vi "FSIS_MAIN.vi"() -> ()   [LabVIEW 2016]
uses:
  <vilib>/FPGAPlugInAG/cRIO-9067/niLvFpga_Open_cRIO-9067.vi
  <vilib>/rvi/interface/common/dynamic/niFpgaDynamicAddResources.vi
  <vilib>/FPGAPlugInAG/Dynamic/niLvFpga_Run_Dynamic.vi
  <vilib>/Utility/file.llb/Read Delimited Spreadsheet (string).vi
  <vilib>/Utility/error.llb/Error Cluster From Error Code.vi
  <vilib>/rvi/errors/niLvFpgaAdjustHostInterfaceError.vi
  <vilib>/FPGAPlugInAG/Dynamic/niLvFpga_Close_Dynamic.vi
  <vilib>/rvi/interface/nirviOpenFPGA/nirviOpenFPGA.xnode
  FPGA Bitfiles/LabVIEWFPGAtests_FPGATarget_SSFPGADrop1_0hIPb3YkEpA.lvbitx
  SS_FPGA_Drop1.vi
  <vilib>/rvi/interface/nirviMethod/nirviMethod.xnode
  <vilib>/rvi/interface/nirviReadWriteControl/nirviReadWriteControl.xnode
  <vilib>/rvi/interface/nirviCloseFPGA/nirviCloseFPGA.xnode
  <vilib>/rvi/interface/Simulation/niFpgaSimulationCallBeginRW.vi
  NiFpgaLv.dll
panel:
  in  "Tab Control":T1(tab)=enum."OPC UA Server"
  in  "millisecond multiple":u32=1000
  in  "INIT Cluster":T2={"Drop1 Address"="172.22.11.2", "Setup FIle Directory"=path "C:/Users/dhomf/Desktop/Schedules/INI_Files", "System"="SS"}
  out "Flow \nMonitoring\nError":errorcluster
  out "Flow Information":T3(array[cluster])=[{"ID"=193, "Channel Information"="SS_2_6_00__COOL_SBF_01", "Channel Name"="1", "Available Flow"=33.2, "No Operations"=25.0, "Good to Operate"=30.0, "M"=193.0, "c"=-10.0}, {"ID"=195, "Channel Information"="SS_2_6_02__COOL_G1F_01", "Channel Name"="1", "Available Flow"=26.5, "No Operations"=20.0, "Good to Operate"=25.0, "M"=195.0, "c"=-10.0}, {"ID"=197, "Channel Information"="SS_2_6_04__COOL_G2F_01", "Channel Name"="1", "Available Flow"=26.5, "No Operations"=15.0, "Good to Operate"=20.0, "M"=197.0, "c"=-10.0}, {"ID"=199, "Channel Information"="SS_2_6_06__COOL_G3F_01", "Channel Name"="1", "Available Flow"=26.5, "No Operations"=20.0, "Good to Operate"=25.0, "M"=199.0, "c"=-10.0}, {"ID"=201, "Channel Information"="SS_2_6_08__COOL_G4F_01", "Channel Name"="1", "Available Flow"=26.5, "No Operations"=20.0, "Good to Operate"=25.0, "M"=201.0, "c"=-10.0}, {"ID"=203, "Channel Information"="SS_2_6_10__COOL_2NF_01", "Channel Name"="1", "Available Flow"=50.5, "No Operations"=38.0, "Good to Operate"=45.0, "M"=203.0, "c"=-10.0}, {"ID"=205, "Channel Information"="SS_2_6_12__COOL_PBF_01", "Channel Name"="1", "Available Flow"=60.0, "No Operations"=52.0, "Good to Operate"=60.0, "M"=205.0, "c"=-25.0}, {"ID"=207, "Channel Information"="SS_2_6_14__COOL_DSF_01", "Channel Name"="1", "Available Flow"=13.8, "No Operations"=10.0, "Good to Operate"=15.0, "M"=207.0, "c"=-10.0}, {"ID"=209, "Channel Information"="SS_2_7_00__COOL_TRF_01", "Channel Name"="1", "Available Flow"=12.0, "No Operations"=8.0, "Good to Operate"=12.0, "M"=209.0, "c"=-10.0}, {"ID"=211, "Channel Information"="SS_2_7_02__COOL_BCF_01", "Channel Name"="1", "Available Flow"=20.5, "No Operations"=12.0, "Good to Operate"=18.0, "M"=211.0, "c"=-10.0}, {"ID"=213, "Channel Information"="SS_2_7_04__COOL_BPF_01", "Channel Name"="1", "Available Flow"=12.0, "No Operations"=8.0, "Good to Operate"=12.0, "M"=213.0, "c"=-10.0}, {"ID"=215, "Channel Information"="SS_2_7_06__COOL_GBF_01", "Channel Name"="1", "Available Flow"=13.8, "No Operations"=8.0, "Good to Operate"=12.0, "M"=215.0, "c"=-10.0}, {"ID"=217, "Channel Information"="SS_2_7_08__COOL_GCF_01", "Channel Name"="1", "Available Flow"=13.8, "No Operations"=8.0, "Good to Operate"=12.0, "M"=217.0, "c"=-10.0}, {"ID"=219, "Channel Information"="SS_2_7_10__COOL_ISF_01", "Channel Name"="1", "Available Flow"=13.8, "No Operations"=10.0, "Good to Operate"=15.0, "M"=219.0, "c"=-10.0}, {"ID"=221, "Channel Information"="SS_2_7_12__COOL_FRF_01", "Channel Name"="1", "Available Flow"=666.0, "No Operations"=540.0, "Good to Operate"=600.0, "M"=221.0, "c"=-298.80478}, {"ID"=222, "Channel Information"="SS_2_7_13__COOL_FEF_01", "Channel Name"="1", "Available Flow"=1350.0, "No Operations"=1250.0, "Good to Operate"=1350.0, "M"=222.0, "c"=-1363.63636}, {"ID"=223, "Channel Information"="SS_2_7_14__COOL_CAF_01", "Channel Name"="1", "Available Flow"=1500.0, "No Operations"=1380.0, "Good to Operate"=1500.0, "M"=223.0, "c"=-1363.63636}]
  out "FPGA Drop1 Reference Error":errorcluster
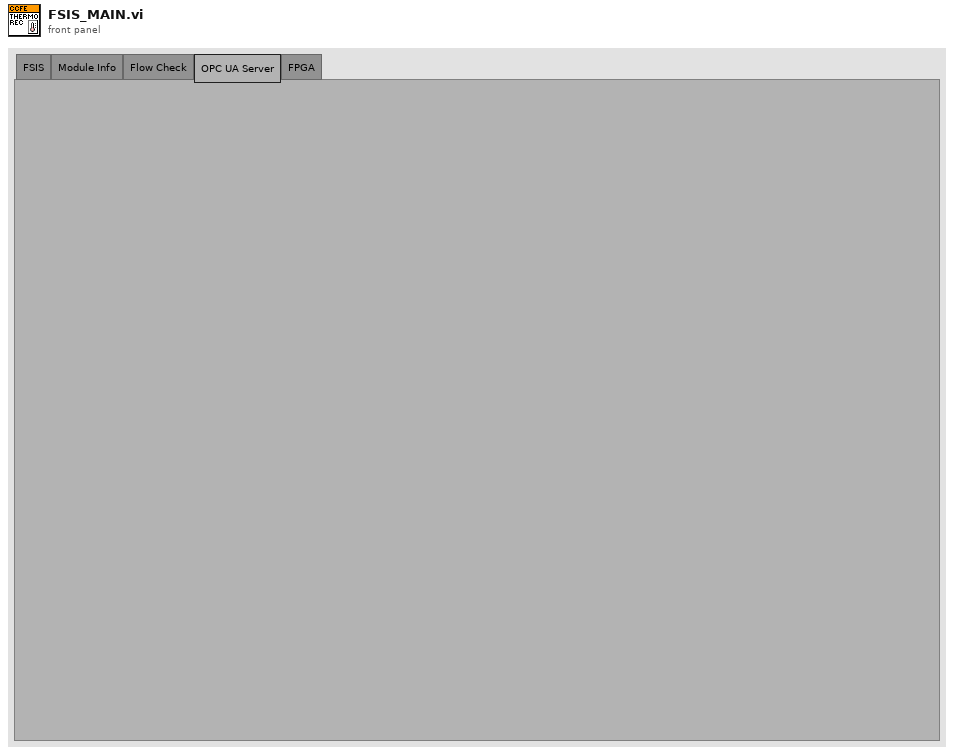
[diagram p1: front panel]
types:
  T1 = enum32{"FSIS", "Module Info", "Flow Check", "OPC UA Server", "FPGA"}
  T2 = cluster{"Drop1 Address":string, "Setup FIle Directory":path, "System":string}
  T3 = cluster{"ID":i32, "Channel Information":string, "Channel Name":string, "Available Flow":dbl, "No Operations":dbl, "Good to Operate":dbl, "M":dbl, "c":dbl}[]
  T4 = cluster{"ID":i32, "Channel Information":string, "Channel Name":string, "Available Flow":dbl, "No Operations":dbl, "Good to Operate":dbl, "M":dbl, "c":dbl}
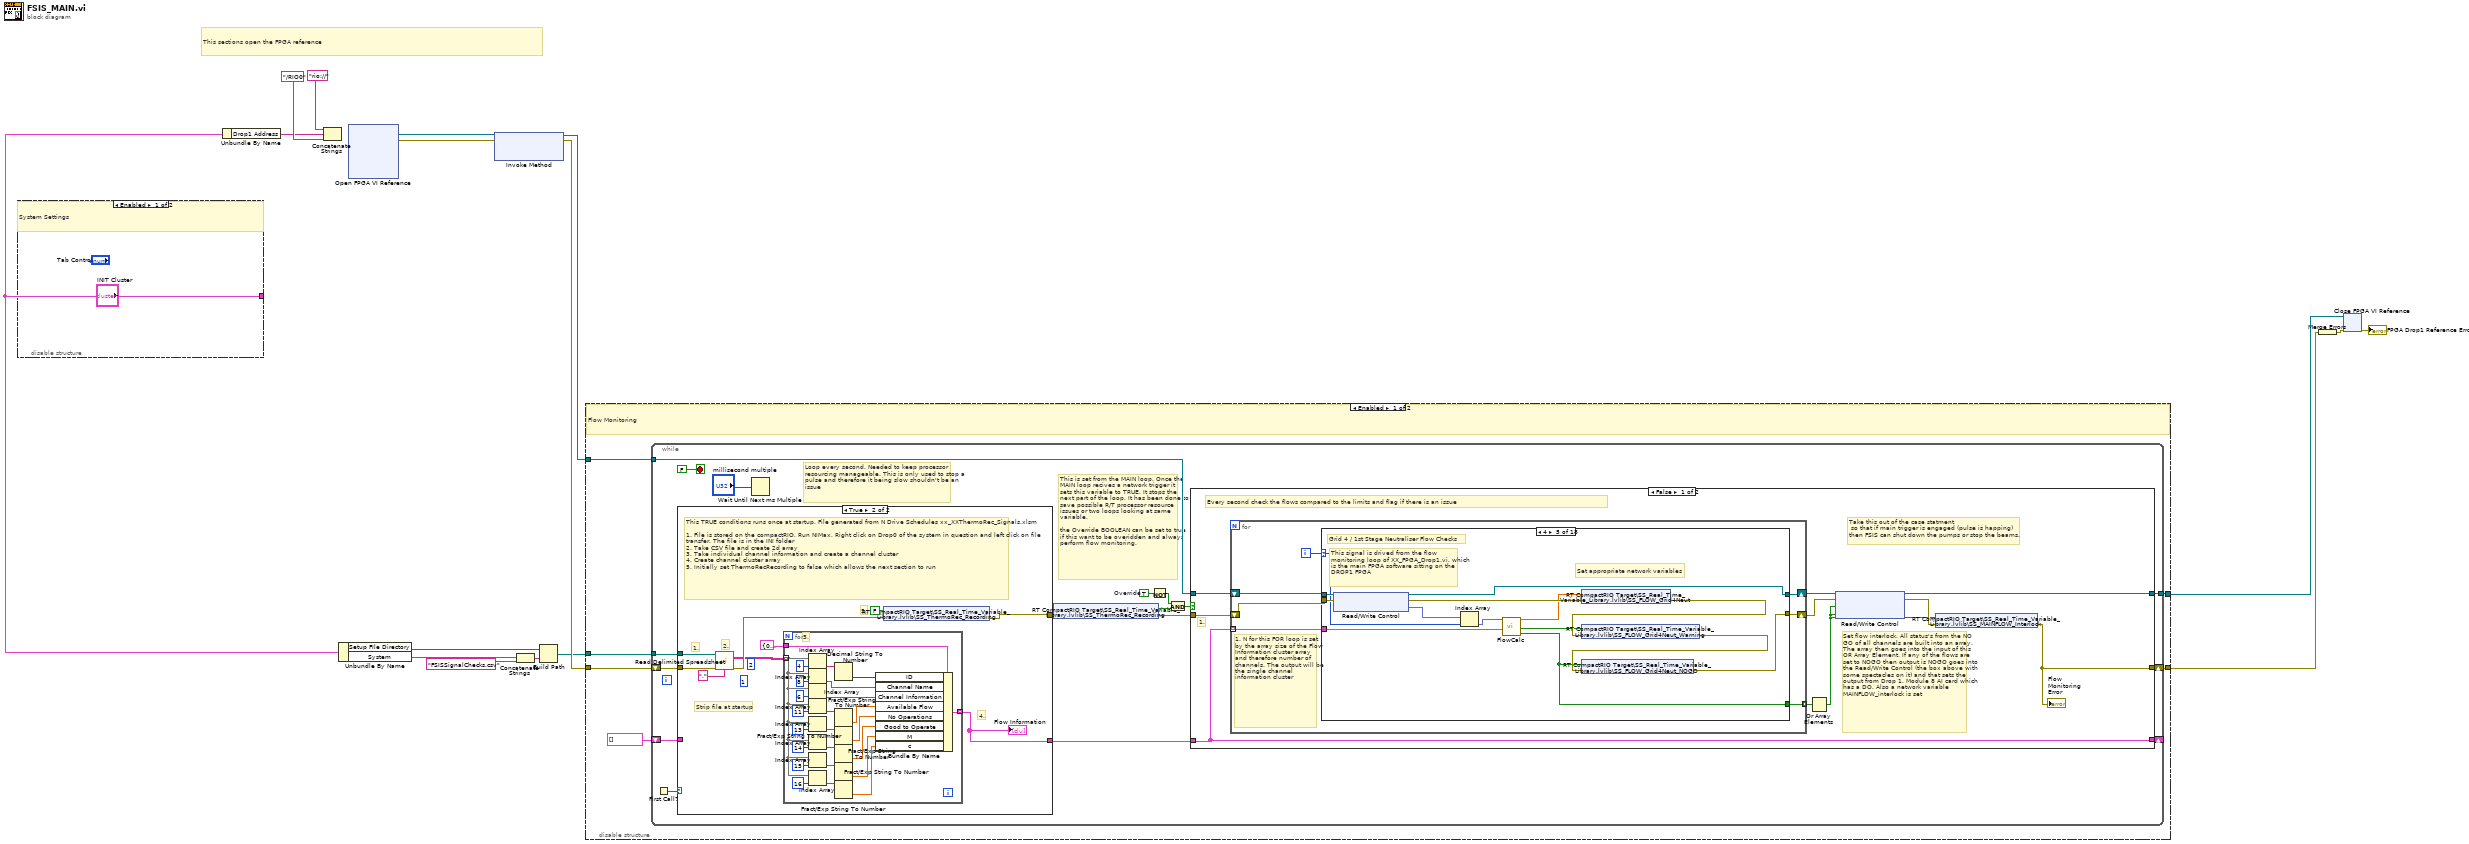
[diagram p0: block diagram]
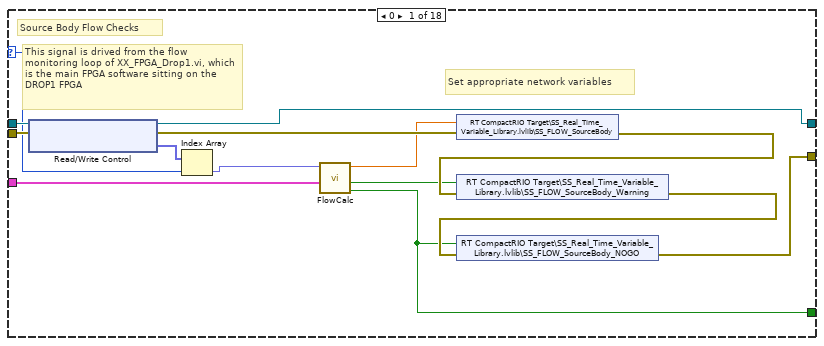
[diagram p3: hidden frame]
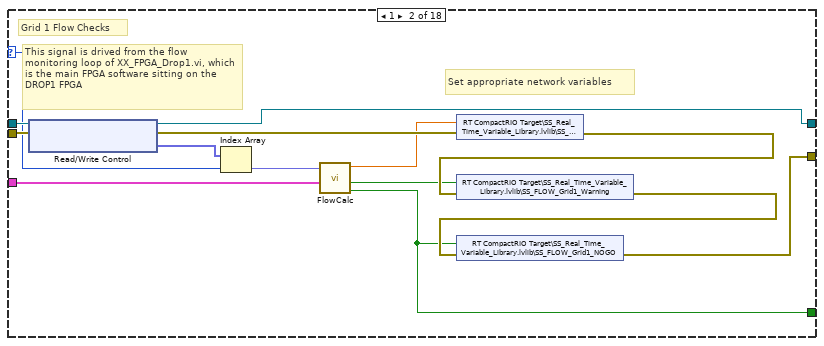
[diagram p4: hidden frame]
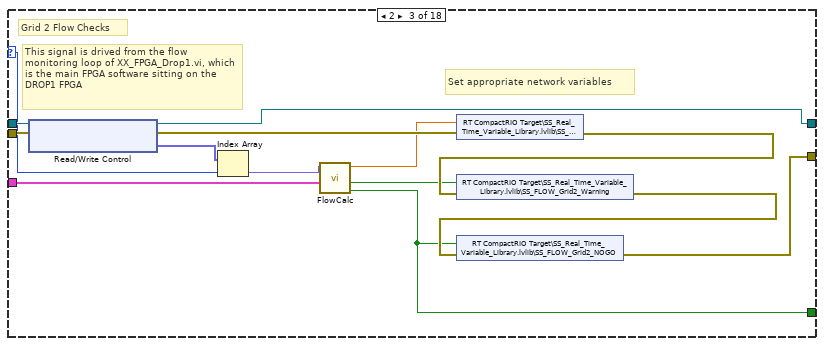
[diagram p5: hidden frame]
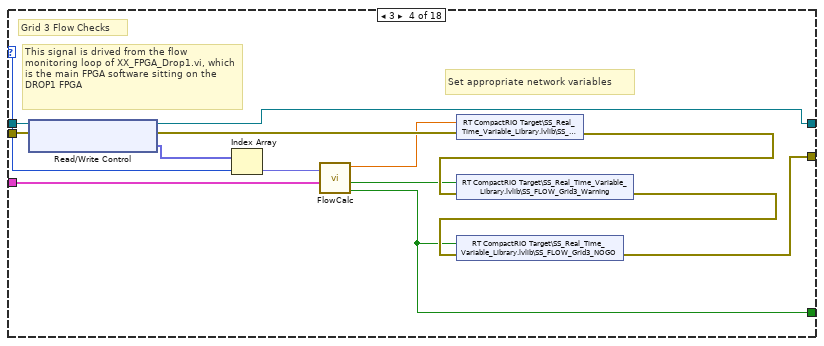
[diagram p6: hidden frame]
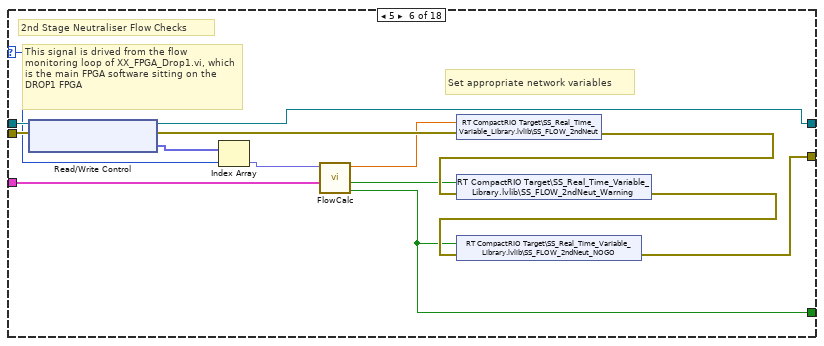
[diagram p7: hidden frame]
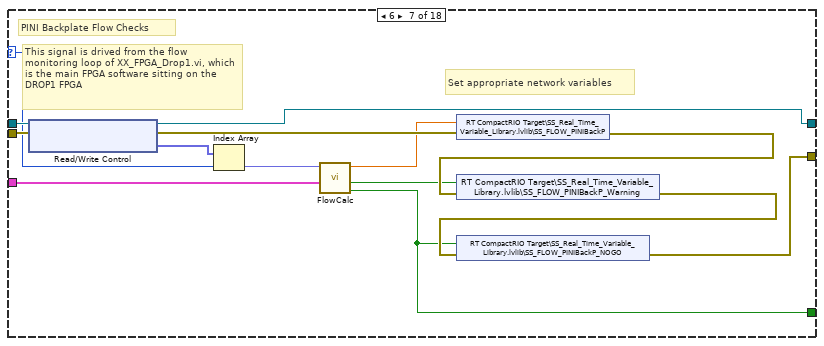
[diagram p8: hidden frame]
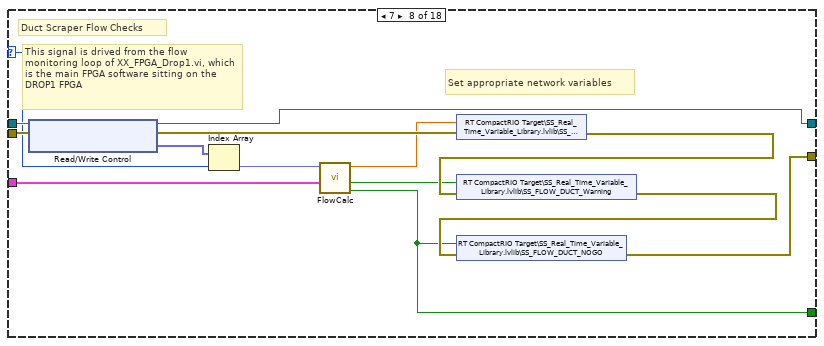
[diagram p9: hidden frame]
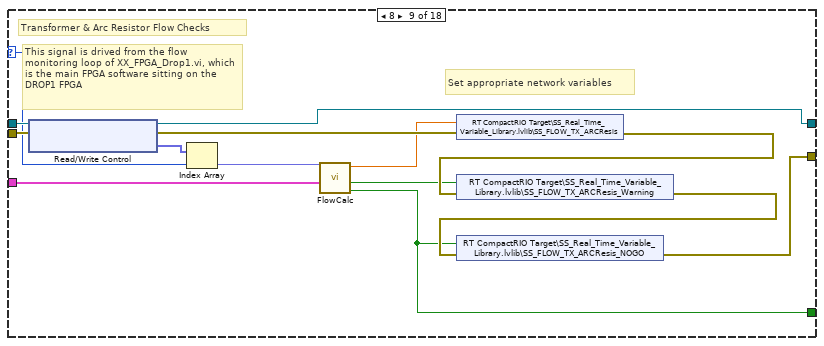
[diagram p10: hidden frame]
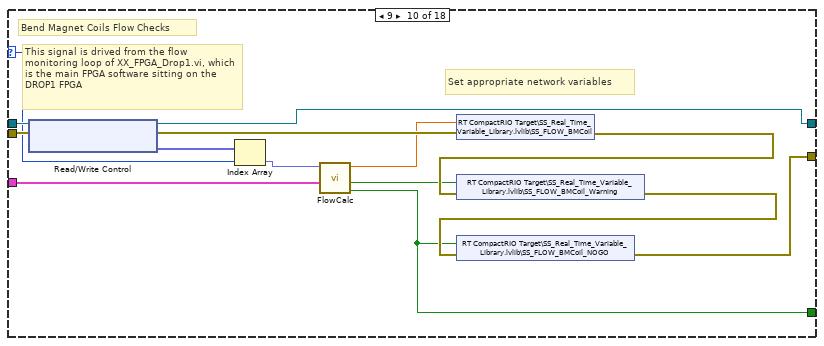
[diagram p11: hidden frame]
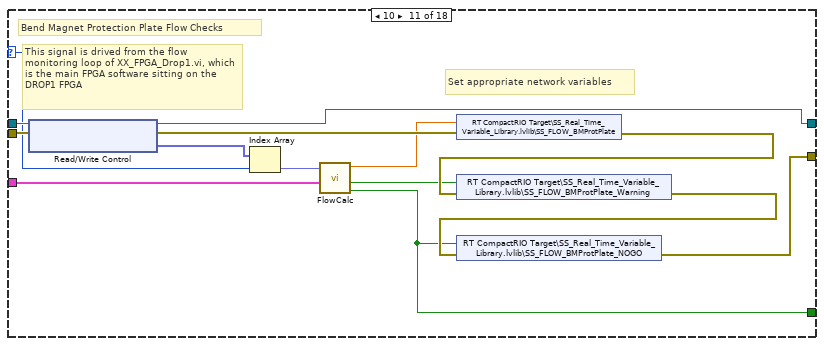
[diagram p12: hidden frame]
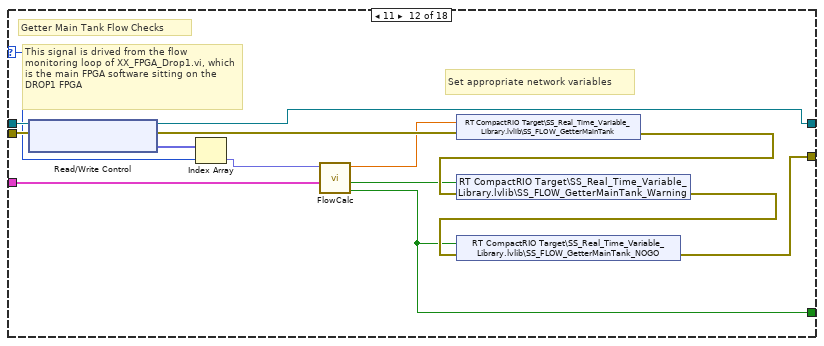
[diagram p13: hidden frame]
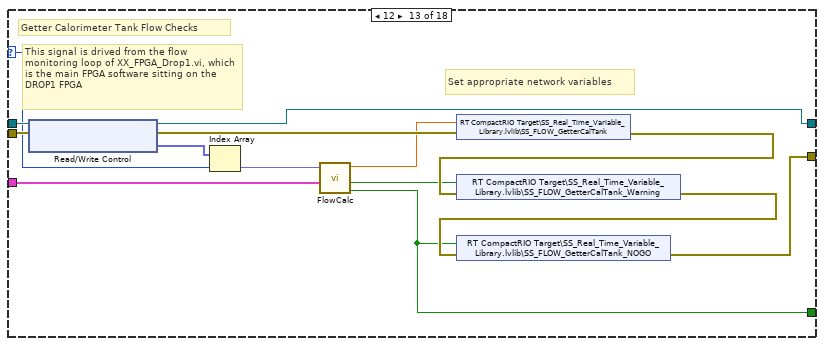
[diagram p14: hidden frame]
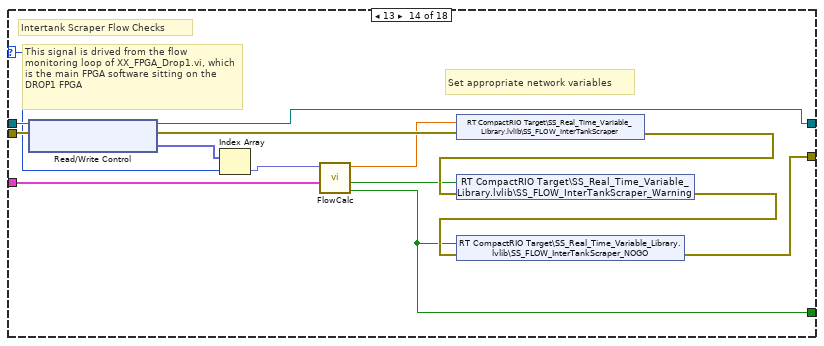
[diagram p15: hidden frame]
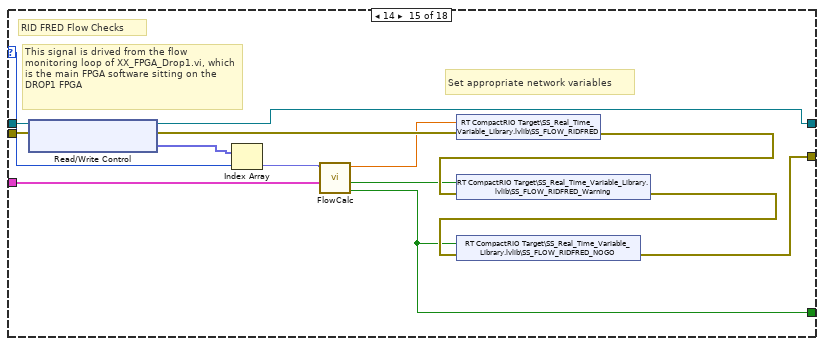
[diagram p16: hidden frame]
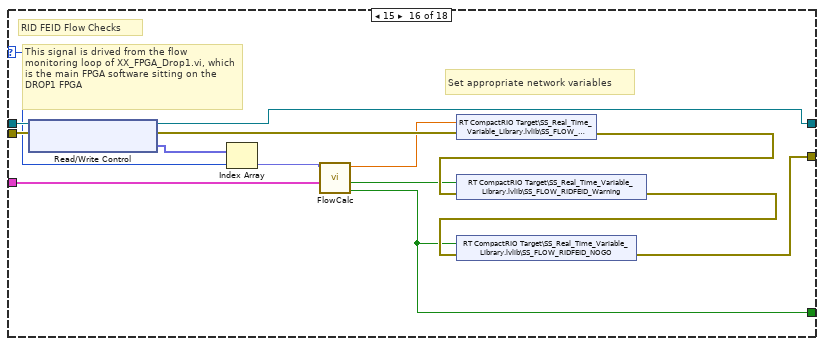
[diagram p17: hidden frame]
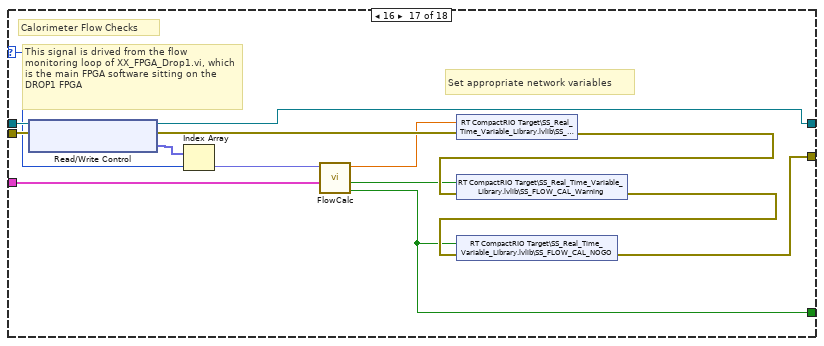
[diagram p18: hidden frame]
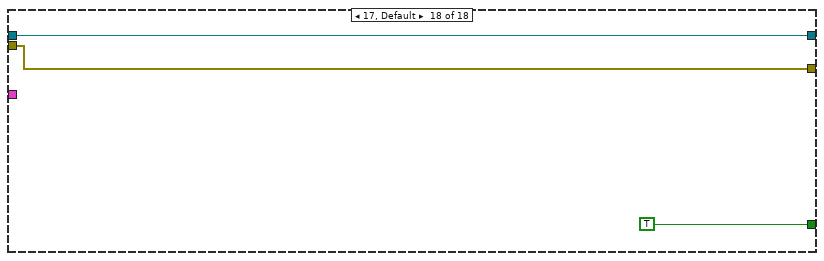
[diagram p19: hidden frame]
diagram:
  # "This sections open the FPGA reference"
  n1 = disable-structure shown="Enabled" {
    disable-tunnel: ["INIT Cluster" _] -> w1
    frame Enabled {
      # "System Settings"
    }
    frame Disabled {
    }
  }
  n2 = Unbundle By Name(w1) -> ("Drop1 Address"=w2:string)
  n3 = Concatenate Strings("rio://", w2, "/RIO0") -> ()  [unwired: 1 out]
  n4 = Unbundle By Name(w1) -> ("Setup FIle Directory"=w4:path, "System"=w3:string)
  n5 = xnode "Open FPGA VI Reference"() -> ("FPGA VI Reference Out"=w14:refnum<k20>, "error out"=w13:errorcluster)  [unwired: 2 in]
  n6 = xnode "Invoke Method"("FPGA VI Reference In"=w14, "error in"=w13) -> ("FPGA VI Reference Out"=w12:refnum<k20>, "error out"=w11:errorcluster)  [unwired: 1 in]
  n7 = Concatenate Strings(w3, "FSISSignalChecks.csv") -> (w7:string)
  n8 = Build Path(base path=w4, name or relative path=w7) -> (appended path=w5:path)
  n9 = disable-structure shown="Enabled" {
    disable-tunnel: [w24 w340] -> w17
    disable-tunnel: w12 -> [w22 w340]
    disable-tunnel: w11 -> [w21 w339]
    disable-tunnel: w5 -> [w20 _]
    disable-tunnel: [w19 w339] -> w8
    frame Enabled {
      # "Flow Monitoring"
      n10 = while {
        shift-right: [w38] -> _
        shift-left: T3 [] ("Flow Information 2") -> [w40]
        tunnel: w22 -> [w36]
        tunnel: [w32] -> w24
        tunnel: w20 -> [w27]
        shift-right: [w26] -> w19
        shift-left: w21 -> [w34]
        stop <- FALSE stop-if-true
        w30 = TRUE  # Override
        # "This is set from the MAIN loop. Once the MAIN loop recives a network trigger it sets this variable to TRUE. It stops the next part of the loop. It has been done to save possible R/T processor resource issues or two loops looking at same variable. \n\nthe Override BOOLEAN can be set to true if this want to be overidden and always perform flow monitoring."
        # "Loop every second. Needed to keep processor resourcing manageable. This is only used to stop a pulse and therefore it being slow shouldn't be an issue"
        # "Flow Monitoring"
        n11 = First Call?() -> (First Call?: T/F=w41:bool)
        n12 = case shown="True" w41 {
          tunnel: w40 -> [w304 _]
          tunnel: [w304 w312] -> w37
          tunnel: w34 -> [w303 w307]
          tunnel: [w303 w308] -> w33
          tunnel: w27 -> [_ w306]
          frame False {
            # "This is the normal situation (after the first loop after startup).  This just passes the information through the FALSE case"
          }
          frame True {
            (unwired) 1 ("index (row)")
            (unwired) 2 ("length")
            # "1."
            # "5."
            # "4."
            # "2."
            # "This TRUE conditions runs once at startup. File generated from N Drive Schedules xx_XXThermoRec_Signals.xlsm\n\n1. File is stored on the compactRIO. Run NIMax, Right click on Drop0 of the system in question and left click on file transfer. The file is in the INI folder\n2. Take CSV file and create 2d array\n3. Take individual channel information and create a channel cluster \n4. Create channel cluster array\n5. Initially set ThermoRecRecording to false which allows the next section to run"
            # "Strip file at startup"
            n13 = call-poly <vilib>:"Read Delimited Spreadsheet.vi"("file path (dialog if empty)"=w306, "error in (no error)"=w307, "delimiter (\\t)"="," ("delimiter (\\t)")) -> ("all rows"=w305:string[][], "error out"=w309:errorcluster)  [unwired: 7 in, 4 out]
            n14 = for {
              tunnel: w305 -> [w317] mode=indexing
              tunnel: T4 {"ID"=0, "Channel Information"="", "Channel Name"="", "Available Flow"=0.0, "No Operations"=0.0, "Good to Operate"=0.0, "M"=0.0, "c"=0.0} ("Flow Information 2") -> [w338]
              tunnel: [w321] -> w312 mode=indexing
              # "3."
              n15 = Index Array(array=w317, index=4) -> (element=w336:string)
              n16 = Index Array(array=w317, index=8) -> (element=w329:string)
              n17 = Index Array(array=w317, index=6) -> (element=w328:string)
              n18 = Index Array(array=w317, index=11) -> (element=w327:string)
              n19 = Index Array(array=w317, index=13) -> (element=w323:string)
              n20 = Index Array(array=w317, index=14) -> (element=w322:string)
              n21 = Index Array(array=w317, index=15) -> (element=w319:string)
              n22 = Index Array(array=w317, index=16) -> (element=w320:string)
              n23 = Fract/Exp String To Number(string=w327) -> (number=w326:dbl)  [unwired: 3 in, 1 out]
              n24 = Fract/Exp String To Number(string=w323) -> (number=w325:dbl)  [unwired: 3 in, 1 out]
              n25 = Fract/Exp String To Number(string=w322) -> (number=w324:dbl)  [unwired: 3 in, 1 out]
              n26 = Fract/Exp String To Number(string=w319) -> (number=w316:dbl)  [unwired: 3 in, 1 out]
              n27 = Fract/Exp String To Number(string=w320) -> (number=w315:dbl)  [unwired: 3 in, 1 out]
              n28 = Decimal String To Number(string=w336) -> (number=w335:i32)  [unwired: 2 in, 1 out]
              n29 = Bundle By Name(cluster=w338, "ID"=w335, "Channel Name"=w329, "Channel Information"=w328, "Available Flow"=w326, "No Operations"=w325, "Good to Operate"=w324, "M"=w316, "c"=w315) -> (w321:T4)
            }
            "Flow Information" <- w312
            n30 = shared-variable "RT CompactRIO Target\\SS_Real_Time_Variable_Library.lvlib\\SS_ThermoRec_Recording"(FALSE ("SS_ThermoRec_Recording"), error in=w309) -> (error out=w308:errorcluster)
          }
        }
        n31 = Wait Until Next ms Multiple(millisecond multiple="millisecond multiple") -> ()  [unwired: 1 out]
        n32 = shared-variable "RT CompactRIO Target\\SS_Real_Time_Variable_Library.lvlib\\SS_ThermoRec_Recording"(error in=w33) -> (w28:bool, error out=w35:errorcluster)
        n33 = Not(x=w30) -> (.not. x?=w31:bool)
        n34 = And(x=w31, y=w28) -> (x .and. y?=w29:bool)
        n35 = case shown="False" w29 {
          tunnel: w37 -> [w45 w302]
          tunnel: [w45 w302] -> w38
          tunnel: w36 -> [w51 w301]
          tunnel: w35 -> [w50 w300]
          tunnel: [w46 w301] -> w32
          tunnel: [w43 w300] -> w26
          frame False {
            # "Take this out of the case statment\n so that if main trigger is engaged (pulse is happing) \nthen FSIS can shut down the pumps or stop the beams."
            # "Set flow interlock. All status's from the NO GO of all channels are built into an array. The array then goes into the input of this OR Array Element. If any of the flows are set to NOGO then output is NOGO goes into the Read/Write Control (the box above with some spectacles on it) and that sets the output from Drop 1, Module 8 AI card which has a DO. Also a network variable MAINFLOW_interlock is set"
            # "1."
            # "Every second check the flows compared to the limits and flag if there is an issue"
            n36 = for {
              tunnel: w45 -> [w52] mode=indexing
              shift-right: [w54] -> w47
              shift-left: w50 -> [w56]
              shift-right: [w55] -> w48
              shift-left: w51 -> [w57]
              tunnel: [w53] -> w49 mode=indexing
              i -> [w58]
              # "1. N for this FOR loop is set by the array size of the Flow Information cluster array and therefore number of channels. The output will be the single channel information cluster"
              n37 = case shown="4" w58 {
                selector: w58 -> [w60 w74 w88 w102 w116 w130 w144 w158 w171 w185 w199 w213 w227 w241 w256 w270 w284 _]
                tunnel: w57 -> [w72 w86 w100 w114 w128 w142 w156 w170 w184 w198 w212 w226 w240 w254 w268 w282 w296 w298]
                tunnel: w56 -> [w71 w85 w99 w113 w127 w141 w155 w169 w183 w197 w211 w225 w239 w253 w267 w281 w295 w299]
                tunnel: [w66 w80 w94 w108 w122 w136 w150 w164 w178 w192 w206 w220 w234 w248 w262 w276 w290 w298] -> w55
                tunnel: [w69 w83 w97 w111 w125 w139 w153 w167 w181 w195 w209 w223 w237 w251 w265 w279 w293 w299] -> w54
                tunnel: [w63 w77 w91 w105 w119 w133 w147 w161 w175 w189 w203 w217 w231 w245 w259 w273 w287 TRUE] -> w53
                tunnel: w52 -> [w65 w79 w93 w107 w121 w135 w149 w163 w177 w191 w205 w219 w233 w247 w261 w275 w289 _]
                frame 0 {
                  # "Set appropriate network variables"
                  # "This signal is drived from the flow monitoring loop of XX_FPGA_Drop1.vi, which is the main FPGA software sitting on the DROP1 FPGA"
                  # "Source Body Flow Checks"
                  n38 = xnode "Read/Write Control"("FPGA VI Reference In"=w72, "error in"=w71) -> ("FPGA VI Reference Out"=w66:refnum<k20>, "error out"=w70:errorcluster, "Raw Data out Mod 1"=w61:fxp<+/-,24,-4>[])
                  n39 = Index Array(array=w61, index=w60) -> (element=w59:fxp<+/-,24,-4>)
                  n40 = call "FlowCalc.vi"("Individual Channel Cluster"=w65, "Flow"=w59) -> ("Flow - No Operations"=w63:bool, "Flow - Warning"=w62:bool, "Flow Rate"=w64:dbl)  [unwired: 7 in]
                  n41 = shared-variable "RT CompactRIO Target\\SS_Real_Time_Variable_Library.lvlib\\SS_FLOW_SourceBody"(w64, error in=w70) -> (error out=w67:errorcluster)
                  n42 = shared-variable "RT CompactRIO Target\\SS_Real_Time_Variable_Library.lvlib\\SS_FLOW_SourceBody_Warning"(w62, error in=w67) -> (error out=w68:errorcluster)
                  n43 = shared-variable "RT CompactRIO Target\\SS_Real_Time_Variable_Library.lvlib\\SS_FLOW_SourceBody_NOGO"(w63, error in=w68) -> (error out=w69:errorcluster)
                }
                frame 1 {
                  # "Grid 1 Flow Checks"
                  # "Set appropriate network variables"
                  # "This signal is drived from the flow monitoring loop of XX_FPGA_Drop1.vi, which is the main FPGA software sitting on the DROP1 FPGA"
                  n44 = xnode "Read/Write Control"("FPGA VI Reference In"=w86, "error in"=w85) -> ("FPGA VI Reference Out"=w80:refnum<k20>, "error out"=w84:errorcluster, "Raw Data out Mod 1"=w75:fxp<+/-,24,-4>[])
                  n45 = Index Array(array=w75, index=w74) -> (element=w73:fxp<+/-,24,-4>)
                  n46 = call "FlowCalc.vi"("Individual Channel Cluster"=w79, "Flow"=w73) -> ("Flow - No Operations"=w77:bool, "Flow - Warning"=w76:bool, "Flow Rate"=w78:dbl)  [unwired: 7 in]
                  n47 = shared-variable "RT CompactRIO Target\\SS_Real_Time_Variable_Library.lvlib\\SS_FLOW_Grid1"(w78, error in=w84) -> (error out=w81:errorcluster)
                  n48 = shared-variable "RT CompactRIO Target\\SS_Real_Time_Variable_Library.lvlib\\SS_FLOW_Grid1_Warning"(w76, error in=w81) -> (error out=w82:errorcluster)
                  n49 = shared-variable "RT CompactRIO Target\\SS_Real_Time_Variable_Library.lvlib\\SS_FLOW_Grid1_NOGO"(w77, error in=w82) -> (error out=w83:errorcluster)
                }
                frame 2 {
                  # "Grid 2 Flow Checks"
                  # "Set appropriate network variables"
                  # "This signal is drived from the flow monitoring loop of XX_FPGA_Drop1.vi, which is the main FPGA software sitting on the DROP1 FPGA"
                  n50 = xnode "Read/Write Control"("FPGA VI Reference In"=w100, "error in"=w99) -> ("FPGA VI Reference Out"=w94:refnum<k20>, "error out"=w98:errorcluster, "Raw Data out Mod 1"=w89:fxp<+/-,24,-4>[])
                  n51 = Index Array(array=w89, index=w88) -> (element=w87:fxp<+/-,24,-4>)
                  n52 = call "FlowCalc.vi"("Individual Channel Cluster"=w93, "Flow"=w87) -> ("Flow - No Operations"=w91:bool, "Flow - Warning"=w90:bool, "Flow Rate"=w92:dbl)  [unwired: 7 in]
                  n53 = shared-variable "RT CompactRIO Target\\SS_Real_Time_Variable_Library.lvlib\\SS_FLOW_Grid2"(w92, error in=w98) -> (error out=w95:errorcluster)
                  n54 = shared-variable "RT CompactRIO Target\\SS_Real_Time_Variable_Library.lvlib\\SS_FLOW_Grid2_Warning"(w90, error in=w95) -> (error out=w96:errorcluster)
                  n55 = shared-variable "RT CompactRIO Target\\SS_Real_Time_Variable_Library.lvlib\\SS_FLOW_Grid2_NOGO"(w91, error in=w96) -> (error out=w97:errorcluster)
                }
                frame 3 {
                  # "Grid 3 Flow Checks"
                  # "Set appropriate network variables"
                  # "This signal is drived from the flow monitoring loop of XX_FPGA_Drop1.vi, which is the main FPGA software sitting on the DROP1 FPGA"
                  n56 = xnode "Read/Write Control"("FPGA VI Reference In"=w114, "error in"=w113) -> ("FPGA VI Reference Out"=w108:refnum<k20>, "error out"=w112:errorcluster, "Raw Data out Mod 1"=w103:fxp<+/-,24,-4>[])
                  n57 = Index Array(array=w103, index=w102) -> (element=w101:fxp<+/-,24,-4>)
                  n58 = call "FlowCalc.vi"("Individual Channel Cluster"=w107, "Flow"=w101) -> ("Flow - No Operations"=w105:bool, "Flow - Warning"=w104:bool, "Flow Rate"=w106:dbl)  [unwired: 7 in]
                  n59 = shared-variable "RT CompactRIO Target\\SS_Real_Time_Variable_Library.lvlib\\SS_FLOW_Grid3"(w106, error in=w112) -> (error out=w109:errorcluster)
                  n60 = shared-variable "RT CompactRIO Target\\SS_Real_Time_Variable_Library.lvlib\\SS_FLOW_Grid3_Warning"(w104, error in=w109) -> (error out=w110:errorcluster)
                  n61 = shared-variable "RT CompactRIO Target\\SS_Real_Time_Variable_Library.lvlib\\SS_FLOW_Grid3_NOGO"(w105, error in=w110) -> (error out=w111:errorcluster)
                }
                frame 4 {
                  # "Grid 4 / 1st Stage Neutraliser Flow Checks"
                  # "Set appropriate network variables"
                  # "This signal is drived from the flow monitoring loop of XX_FPGA_Drop1.vi, which is the main FPGA software sitting on the DROP1 FPGA"
                  n62 = xnode "Read/Write Control"("FPGA VI Reference In"=w128, "error in"=w127) -> ("FPGA VI Reference Out"=w122:refnum<k20>, "error out"=w126:errorcluster, "Raw Data out Mod 1"=w117:fxp<+/-,24,-4>[])
                  n63 = Index Array(array=w117, index=w116) -> (element=w115:fxp<+/-,24,-4>)
                  n64 = call "FlowCalc.vi"("Individual Channel Cluster"=w121, "Flow"=w115) -> ("Flow - No Operations"=w119:bool, "Flow - Warning"=w118:bool, "Flow Rate"=w120:dbl)  [unwired: 7 in]
                  n65 = shared-variable "RT CompactRIO Target\\SS_Real_Time_Variable_Library.lvlib\\SS_FLOW_Grid4Neut"(w120, error in=w126) -> (error out=w123:errorcluster)
                  n66 = shared-variable "RT CompactRIO Target\\SS_Real_Time_Variable_Library.lvlib\\SS_FLOW_Grid4Neut_Warning"(w118, error in=w123) -> (error out=w124:errorcluster)
                  n67 = shared-variable "RT CompactRIO Target\\SS_Real_Time_Variable_Library.lvlib\\SS_FLOW_Grid4Neut_NOGO"(w119, error in=w124) -> (error out=w125:errorcluster)
                }
                frame 5 {
                  # "2nd Stage Neutraliser Flow Checks"
                  # "Set appropriate network variables"
                  # "This signal is drived from the flow monitoring loop of XX_FPGA_Drop1.vi, which is the main FPGA software sitting on the DROP1 FPGA"
                  n68 = xnode "Read/Write Control"("FPGA VI Reference In"=w142, "error in"=w141) -> ("FPGA VI Reference Out"=w136:refnum<k20>, "error out"=w140:errorcluster, "Raw Data out Mod 1"=w131:fxp<+/-,24,-4>[])
                  n69 = Index Array(array=w131, index=w130) -> (element=w129:fxp<+/-,24,-4>)
                  n70 = call "FlowCalc.vi"("Individual Channel Cluster"=w135, "Flow"=w129) -> ("Flow - No Operations"=w133:bool, "Flow - Warning"=w132:bool, "Flow Rate"=w134:dbl)  [unwired: 7 in]
                  n71 = shared-variable "RT CompactRIO Target\\SS_Real_Time_Variable_Library.lvlib\\SS_FLOW_2ndNeut"(w134, error in=w140) -> (error out=w137:errorcluster)
                  n72 = shared-variable "RT CompactRIO Target\\SS_Real_Time_Variable_Library.lvlib\\SS_FLOW_2ndNeut_Warning"(w132, error in=w137) -> (error out=w138:errorcluster)
                  n73 = shared-variable "RT CompactRIO Target\\SS_Real_Time_Variable_Library.lvlib\\SS_FLOW_2ndNeut_NOGO"(w133, error in=w138) -> (error out=w139:errorcluster)
                }
                frame 6 {
                  # "PINI Backplate Flow Checks"
                  # "Set appropriate network variables"
                  # "This signal is drived from the flow monitoring loop of XX_FPGA_Drop1.vi, which is the main FPGA software sitting on the DROP1 FPGA"
                  n74 = xnode "Read/Write Control"("FPGA VI Reference In"=w156, "error in"=w155) -> ("FPGA VI Reference Out"=w150:refnum<k20>, "error out"=w154:errorcluster, "Raw Data out Mod 1"=w145:fxp<+/-,24,-4>[])
                  n75 = Index Array(array=w145, index=w144) -> (element=w143:fxp<+/-,24,-4>)
                  n76 = call "FlowCalc.vi"("Individual Channel Cluster"=w149, "Flow"=w143) -> ("Flow - No Operations"=w147:bool, "Flow - Warning"=w146:bool, "Flow Rate"=w148:dbl)  [unwired: 7 in]
                  n77 = shared-variable "RT CompactRIO Target\\SS_Real_Time_Variable_Library.lvlib\\SS_FLOW_PINIBackP"(w148, error in=w154) -> (error out=w151:errorcluster)
                  n78 = shared-variable "RT CompactRIO Target\\SS_Real_Time_Variable_Library.lvlib\\SS_FLOW_PINIBackP_Warning"(w146, error in=w151) -> (error out=w152:errorcluster)
                  n79 = shared-variable "RT CompactRIO Target\\SS_Real_Time_Variable_Library.lvlib\\SS_FLOW_PINIBackP_NOGO"(w147, error in=w152) -> (error out=w153:errorcluster)
                }
                frame 7 {
                  # "Duct Scraper Flow Checks"
                  # "Set appropriate network variables"
                  # "This signal is drived from the flow monitoring loop of XX_FPGA_Drop1.vi, which is the main FPGA software sitting on the DROP1 FPGA"
                  n80 = xnode "Read/Write Control"("FPGA VI Reference In"=w170, "error in"=w169) -> ("FPGA VI Reference Out"=w164:refnum<k20>, "error out"=w168:errorcluster, "Raw Data out Mod 1"=w159:fxp<+/-,24,-4>[])
                  n81 = Index Array(array=w159, index=w158) -> (element=w157:fxp<+/-,24,-4>)
                  n82 = call "FlowCalc.vi"("Individual Channel Cluster"=w163, "Flow"=w157) -> ("Flow - No Operations"=w161:bool, "Flow - Warning"=w160:bool, "Flow Rate"=w162:dbl)  [unwired: 7 in]
                  n83 = shared-variable "RT CompactRIO Target\\SS_Real_Time_Variable_Library.lvlib\\SS_FLOW_DUCT"(w162, error in=w168) -> (error out=w165:errorcluster)
                  n84 = shared-variable "RT CompactRIO Target\\SS_Real_Time_Variable_Library.lvlib\\SS_FLOW_DUCT_Warning"(w160, error in=w165) -> (error out=w166:errorcluster)
                  n85 = shared-variable "RT CompactRIO Target\\SS_Real_Time_Variable_Library.lvlib\\SS_FLOW_DUCT_NOGO"(w161, error in=w166) -> (error out=w167:errorcluster)
                }
                frame 8 {
                  # "Transformer & Arc Resistor Flow Checks"
                  # "Set appropriate network variables"
                  # "This signal is drived from the flow monitoring loop of XX_FPGA_Drop1.vi, which is the main FPGA software sitting on the DROP1 FPGA"
                  n86 = xnode "Read/Write Control"("FPGA VI Reference In"=w184, "error in"=w183) -> ("FPGA VI Reference Out"=w178:refnum<k20>, "error out"=w182:errorcluster, "Raw Data out Mod 1"=w172:fxp<+/-,24,-4>[])
                  n87 = Index Array(array=w172, index=w171) -> (element=w173:fxp<+/-,24,-4>)
                  n88 = call "FlowCalc.vi"("Individual Channel Cluster"=w177, "Flow"=w173) -> ("Flow - No Operations"=w175:bool, "Flow - Warning"=w174:bool, "Flow Rate"=w176:dbl)  [unwired: 7 in]
                  n89 = shared-variable "RT CompactRIO Target\\SS_Real_Time_Variable_Library.lvlib\\SS_FLOW_TX_ARCResis"(w176, error in=w182) -> (error out=w179:errorcluster)
                  n90 = shared-variable "RT CompactRIO Target\\SS_Real_Time_Variable_Library.lvlib\\SS_FLOW_TX_ARCResis_Warning"(w174, error in=w179) -> (error out=w180:errorcluster)
                  n91 = shared-variable "RT CompactRIO Target\\SS_Real_Time_Variable_Library.lvlib\\SS_FLOW_TX_ARCResis_NOGO"(w175, error in=w180) -> (error out=w181:errorcluster)
                }
                frame 9 {
                  # "Bend Magnet Coils Flow Checks"
                  # "Set appropriate network variables"
                  # "This signal is drived from the flow monitoring loop of XX_FPGA_Drop1.vi, which is the main FPGA software sitting on the DROP1 FPGA"
                  n92 = xnode "Read/Write Control"("FPGA VI Reference In"=w198, "error in"=w197) -> ("FPGA VI Reference Out"=w192:refnum<k20>, "error out"=w196:errorcluster, "Raw Data out Mod 1"=w186:fxp<+/-,24,-4>[])
                  n93 = Index Array(array=w186, index=w185) -> (element=w187:fxp<+/-,24,-4>)
                  n94 = call "FlowCalc.vi"("Individual Channel Cluster"=w191, "Flow"=w187) -> ("Flow - No Operations"=w189:bool, "Flow - Warning"=w188:bool, "Flow Rate"=w190:dbl)  [unwired: 7 in]
                  n95 = shared-variable "RT CompactRIO Target\\SS_Real_Time_Variable_Library.lvlib\\SS_FLOW_BMCoil"(w190, error in=w196) -> (error out=w193:errorcluster)
                  n96 = shared-variable "RT CompactRIO Target\\SS_Real_Time_Variable_Library.lvlib\\SS_FLOW_BMCoil_Warning"(w188, error in=w193) -> (error out=w194:errorcluster)
                  n97 = shared-variable "RT CompactRIO Target\\SS_Real_Time_Variable_Library.lvlib\\SS_FLOW_BMCoil_NOGO"(w189, error in=w194) -> (error out=w195:errorcluster)
                }
                frame 10 {
                  # "Bend Magnet Protection Plate Flow Checks"
                  # "Set appropriate network variables"
                  # "This signal is drived from the flow monitoring loop of XX_FPGA_Drop1.vi, which is the main FPGA software sitting on the DROP1 FPGA"
                  n98 = xnode "Read/Write Control"("FPGA VI Reference In"=w212, "error in"=w211) -> ("FPGA VI Reference Out"=w206:refnum<k20>, "error out"=w210:errorcluster, "Raw Data out Mod 1"=w200:fxp<+/-,24,-4>[])
                  n99 = Index Array(array=w200, index=w199) -> (element=w201:fxp<+/-,24,-4>)
                  n100 = call "FlowCalc.vi"("Individual Channel Cluster"=w205, "Flow"=w201) -> ("Flow - No Operations"=w203:bool, "Flow - Warning"=w202:bool, "Flow Rate"=w204:dbl)  [unwired: 7 in]
                  n101 = shared-variable "RT CompactRIO Target\\SS_Real_Time_Variable_Library.lvlib\\SS_FLOW_BMProtPlate"(w204, error in=w210) -> (error out=w207:errorcluster)
                  n102 = shared-variable "RT CompactRIO Target\\SS_Real_Time_Variable_Library.lvlib\\SS_FLOW_BMProtPlate_Warning"(w202, error in=w207) -> (error out=w208:errorcluster)
                  n103 = shared-variable "RT CompactRIO Target\\SS_Real_Time_Variable_Library.lvlib\\SS_FLOW_BMProtPlate_NOGO"(w203, error in=w208) -> (error out=w209:errorcluster)
                }
                frame 11 {
                  # "Getter Main Tank Flow Checks"
                  # "Set appropriate network variables"
                  # "This signal is drived from the flow monitoring loop of XX_FPGA_Drop1.vi, which is the main FPGA software sitting on the DROP1 FPGA"
                  n104 = xnode "Read/Write Control"("FPGA VI Reference In"=w226, "error in"=w225) -> ("FPGA VI Reference Out"=w220:refnum<k20>, "error out"=w224:errorcluster, "Raw Data out Mod 1"=w214:fxp<+/-,24,-4>[])
                  n105 = Index Array(array=w214, index=w213) -> (element=w215:fxp<+/-,24,-4>)
                  n106 = call "FlowCalc.vi"("Individual Channel Cluster"=w219, "Flow"=w215) -> ("Flow - No Operations"=w217:bool, "Flow - Warning"=w216:bool, "Flow Rate"=w218:dbl)  [unwired: 7 in]
                  n107 = shared-variable "RT CompactRIO Target\\SS_Real_Time_Variable_Library.lvlib\\SS_FLOW_GetterMainTank"(w218, error in=w224) -> (error out=w221:errorcluster)
                  n108 = shared-variable "RT CompactRIO Target\\SS_Real_Time_Variable_Library.lvlib\\SS_FLOW_GetterMainTank_Warning"(w216, error in=w221) -> (error out=w222:errorcluster)
                  n109 = shared-variable "RT CompactRIO Target\\SS_Real_Time_Variable_Library.lvlib\\SS_FLOW_GetterMainTank_NOGO"(w217, error in=w222) -> (error out=w223:errorcluster)
                }
                frame 12 {
                  # "Getter Calorimeter Tank Flow Checks"
                  # "Set appropriate network variables"
                  # "This signal is drived from the flow monitoring loop of XX_FPGA_Drop1.vi, which is the main FPGA software sitting on the DROP1 FPGA"
                  n110 = xnode "Read/Write Control"("FPGA VI Reference In"=w240, "error in"=w239) -> ("FPGA VI Reference Out"=w234:refnum<k20>, "error out"=w238:errorcluster, "Raw Data out Mod 1"=w228:fxp<+/-,24,-4>[])
                  n111 = Index Array(array=w228, index=w227) -> (element=w229:fxp<+/-,24,-4>)
                  n112 = call "FlowCalc.vi"("Individual Channel Cluster"=w233, "Flow"=w229) -> ("Flow - No Operations"=w231:bool, "Flow - Warning"=w230:bool, "Flow Rate"=w232:dbl)  [unwired: 7 in]
                  n113 = shared-variable "RT CompactRIO Target\\SS_Real_Time_Variable_Library.lvlib\\SS_FLOW_GetterCalTank"(w232, error in=w238) -> (error out=w235:errorcluster)
                  n114 = shared-variable "RT CompactRIO Target\\SS_Real_Time_Variable_Library.lvlib\\SS_FLOW_GetterCalTank_Warning"(w230, error in=w235) -> (error out=w236:errorcluster)
                  n115 = shared-variable "RT CompactRIO Target\\SS_Real_Time_Variable_Library.lvlib\\SS_FLOW_GetterCalTank_NOGO"(w231, error in=w236) -> (error out=w237:errorcluster)
                }
                frame 13 {
                  # "Intertank Scraper Flow Checks"
                  # "Set appropriate network variables"
                  # "This signal is drived from the flow monitoring loop of XX_FPGA_Drop1.vi, which is the main FPGA software sitting on the DROP1 FPGA"
                  n116 = xnode "Read/Write Control"("FPGA VI Reference In"=w254, "error in"=w253) -> ("FPGA VI Reference Out"=w248:refnum<k20>, "error out"=w252:errorcluster, "Raw Data out Mod 1"=w242:fxp<+/-,24,-4>[])
                  n117 = Index Array(array=w242, index=w241) -> (element=w243:fxp<+/-,24,-4>)
                  n118 = call "FlowCalc.vi"("Individual Channel Cluster"=w247, "Flow"=w243) -> ("Flow - No Operations"=w245:bool, "Flow - Warning"=w244:bool, "Flow Rate"=w246:dbl)  [unwired: 7 in]
                  n119 = shared-variable "RT CompactRIO Target\\SS_Real_Time_Variable_Library.lvlib\\SS_FLOW_InterTankScraper"(w246, error in=w252) -> (error out=w249:errorcluster)
                  n120 = shared-variable "RT CompactRIO Target\\SS_Real_Time_Variable_Library.lvlib\\SS_FLOW_InterTankScraper_Warning"(w244, error in=w249) -> (error out=w250:errorcluster)
                  n121 = shared-variable "RT CompactRIO Target\\SS_Real_Time_Variable_Library.lvlib\\SS_FLOW_InterTankScraper_NOGO"(w245, error in=w250) -> (error out=w251:errorcluster)
                }
                frame 14 {
                  # "RID FRED Flow Checks"
                  # "Set appropriate network variables"
                  # "This signal is drived from the flow monitoring loop of XX_FPGA_Drop1.vi, which is the main FPGA software sitting on the DROP1 FPGA"
                  n122 = xnode "Read/Write Control"("FPGA VI Reference In"=w268, "error in"=w267) -> ("FPGA VI Reference Out"=w262:refnum<k20>, "error out"=w266:errorcluster, "Raw Data out Mod 1"=w257:fxp<+/-,24,-4>[])
                  n123 = Index Array(array=w257, index=w256) -> (element=w255:fxp<+/-,24,-4>)
                  n124 = call "FlowCalc.vi"("Individual Channel Cluster"=w261, "Flow"=w255) -> ("Flow - No Operations"=w259:bool, "Flow - Warning"=w258:bool, "Flow Rate"=w260:dbl)  [unwired: 7 in]
                  n125 = shared-variable "RT CompactRIO Target\\SS_Real_Time_Variable_Library.lvlib\\SS_FLOW_RIDFRED"(w260, error in=w266) -> (error out=w263:errorcluster)
                  n126 = shared-variable "RT CompactRIO Target\\SS_Real_Time_Variable_Library.lvlib\\SS_FLOW_RIDFRED_Warning"(w258, error in=w263) -> (error out=w264:errorcluster)
                  n127 = shared-variable "RT CompactRIO Target\\SS_Real_Time_Variable_Library.lvlib\\SS_FLOW_RIDFRED_NOGO"(w259, error in=w264) -> (error out=w265:errorcluster)
                }
                frame 15 {
                  # "RID FEID Flow Checks"
                  # "Set appropriate network variables"
                  # "This signal is drived from the flow monitoring loop of XX_FPGA_Drop1.vi, which is the main FPGA software sitting on the DROP1 FPGA"
                  n128 = xnode "Read/Write Control"("FPGA VI Reference In"=w282, "error in"=w281) -> ("FPGA VI Reference Out"=w276:refnum<k20>, "error out"=w280:errorcluster, "Raw Data out Mod 1"=w271:fxp<+/-,24,-4>[])
                  n129 = Index Array(array=w271, index=w270) -> (element=w269:fxp<+/-,24,-4>)
                  n130 = call "FlowCalc.vi"("Individual Channel Cluster"=w275, "Flow"=w269) -> ("Flow - No Operations"=w273:bool, "Flow - Warning"=w272:bool, "Flow Rate"=w274:dbl)  [unwired: 7 in]
                  n131 = shared-variable "RT CompactRIO Target\\SS_Real_Time_Variable_Library.lvlib\\SS_FLOW_RIDFEID"(w274, error in=w280) -> (error out=w277:errorcluster)
                  n132 = shared-variable "RT CompactRIO Target\\SS_Real_Time_Variable_Library.lvlib\\SS_FLOW_RIDFEID_Warning"(w272, error in=w277) -> (error out=w278:errorcluster)
                  n133 = shared-variable "RT CompactRIO Target\\SS_Real_Time_Variable_Library.lvlib\\SS_FLOW_RIDFEID_NOGO"(w273, error in=w278) -> (error out=w279:errorcluster)
                }
                frame 16 {
                  # "Calorimeter Flow Checks"
                  # "Set appropriate network variables"
                  # "This signal is drived from the flow monitoring loop of XX_FPGA_Drop1.vi, which is the main FPGA software sitting on the DROP1 FPGA"
                  n134 = xnode "Read/Write Control"("FPGA VI Reference In"=w296, "error in"=w295) -> ("FPGA VI Reference Out"=w290:refnum<k20>, "error out"=w294:errorcluster, "Raw Data out Mod 1"=w285:fxp<+/-,24,-4>[])
                  n135 = Index Array(array=w285, index=w284) -> (element=w283:fxp<+/-,24,-4>)
                  n136 = call "FlowCalc.vi"("Individual Channel Cluster"=w289, "Flow"=w283) -> ("Flow - No Operations"=w287:bool, "Flow - Warning"=w286:bool, "Flow Rate"=w288:dbl)  [unwired: 7 in]
                  n137 = shared-variable "RT CompactRIO Target\\SS_Real_Time_Variable_Library.lvlib\\SS_FLOW_CAL"(w288, error in=w294) -> (error out=w291:errorcluster)
                  n138 = shared-variable "RT CompactRIO Target\\SS_Real_Time_Variable_Library.lvlib\\SS_FLOW_CAL_Warning"(w286, error in=w291) -> (error out=w292:errorcluster)
                  n139 = shared-variable "RT CompactRIO Target\\SS_Real_Time_Variable_Library.lvlib\\SS_FLOW_CAL_NOGO"(w287, error in=w292) -> (error out=w293:errorcluster)
                }
                frame 17, Default {
                }
              }
            }
            n140 = Or Array Elements(Boolean array=w49) -> (logical OR=w42:bool)
            n141 = xnode "Read/Write Control"("FPGA VI Reference In"=w48, "error in"=w47, "Set Flow Interlock"=w42, "Set Pump Interlock"=w42) -> ("FPGA VI Reference Out"=w46:refnum<k20>, "error out"=w44:errorcluster)
            n142 = shared-variable "RT CompactRIO Target\\SS_Real_Time_Variable_Library.lvlib\\SS_MAINFLOW_Interlock"(w42, error in=w44) -> (error out=w43:errorcluster)
            "Flow \nMonitoring\nError" <- w43
          }
          frame True {
            # "A pulse is running stop monitoring until after the pulse. The flows will be recorded in the pulse file anyway"
          }
        }
      }
    }
    frame Disabled {
      # "Flow Monitoring Disabled"
    }
  }
  n143 = Merge Errors(w8) -> (w15:errorcluster)
  n144 = xnode "Close FPGA VI Reference"("FPGA VI Reference In"=w17, "error in"=w15) -> ("error out"=→"FPGA Drop1 Reference Error":errorcluster)
